vi "IntakeGlobal.vi"() -> ()   [LabVIEW 2023]
doc: "Holds intake globals:\n--MotorDemandTop--numeric\n--MotorDemandLeft--numeric\n--MotorDemandRight--numeric\n--HaveCoralSensor--boolean\n--HaveAlgaeSensor--boolean"
uses:
  IntakeStates.ctl
panel:
  out "Debug_CancelCount":i32
  out "Debug_DepAlgaeCount":i32
  out "Debug_DepCoralCount":i32
  out "Debug_AlgaeCount":i32
  out "Debug_CoralCount":i32
  out "CurrentState":T1
  in  "HaveAlgaeSensor":bool
  in  "HaveCoralSensor":bool
  out "MotorDemandRight":dbl
  out "MotorDemandLeft":dbl
  out "MotorDemandTop":dbl
  # "COMMAND DEBUG"
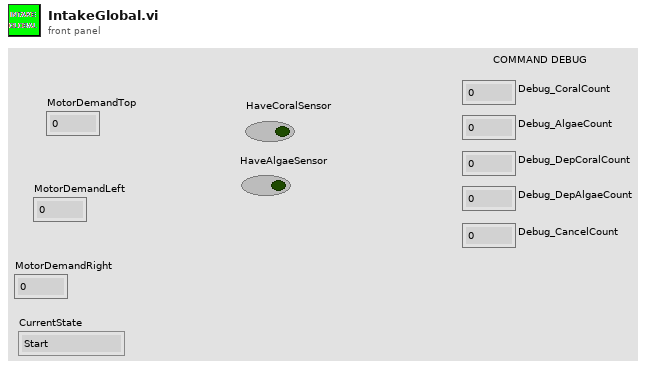
[diagram p1: front panel]
types:
  T1 = typedef "IntakeStates.ctl" = enum16{"Start", "WaitForCommand", "IntakeCoral", "IntakeAlgae", "WaitForCoral", "WaitForAlgae", "DepositCoral", "DepositAlgae", "DepositCoralTimer", "DepositAlgaeTimer"}
diagram:
